vi "Cancella Celle.vi"(0 "report in":T1, 7 "start (-1, -1)":cluster{"row":i32, "column":i32}={"row"=-1, "column"=-1}, 9 "end (-1, -1)":cluster{"row":i32, "column":i32}={"row"=-1, "column"=-1}, 11 "error in (no error)":errorcluster, 12 "name (\"\")":string) -> (4 "report out":T1, 15 "error out":errorcluster)   [LabVIEW 2022 SP3]
doc: "Merges the range of cells specified by the start and end clusters."
uses:
  <vilib>/Utility/NIReport.llb/NI_ReportGenerationCore.lvlib
  <vilib>/Utility/NIReport.llb/NI_report.lvclass
  <vilib>/Utility/NIReport.llb/Generate Report Object Reference.ctl
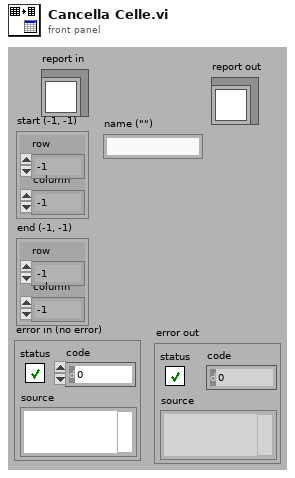
[diagram p1: front panel]
types:
  T1 = typedef "Generate Report Object Reference.ctl" = refnum<class "NI_report.lvclass">
  T2 = typedef "Generate Report Data Members.ctl" = cluster{"Title Text":string, "Header Text":string, "Body Text":string, "Footer Text":string, "Image List":path[], "NIReports.Report":refnum<k7>, "Report Type":enum16{"Standard Report", "HTML", "Word", "Excel"}, "Font Tag":string, "Word._Application":refnum<k7>, "Word._Document":refnum<k7>, "Word.Documents":refnum<k7>, "Word.InlineShapes":refnum<k7>, "Word.Tables":refnum<k7>, "Excel._Application":refnum<k7>, "Excel._Workbook":refnum<k7>, "Excel._Worksheet":refnum<k7>, "Excel.Sheets":refnum<k7>, "Excel.Shapes":refnum<k7>, "font":T3, "application directory":path}
  T3 = typedef "font.ctl" = cluster{"font name":string, "font size":dbl, "bold":u16, "italic":u16, "underline":u16, "strike through":u16, "font color":u32}
  T4 = typedef "Generate Report Object Reference.ctl" = refnum<k1>
  T5 = enum16{"Standard Report", "HTML", "Word", "Excel"}
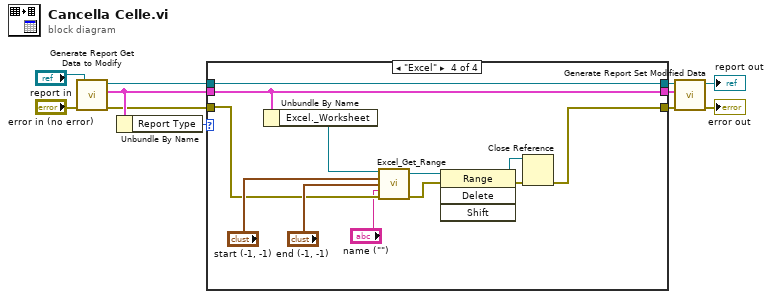
[diagram p0: block diagram]
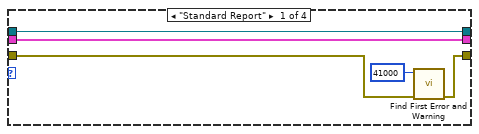
[diagram p2: hidden frame]
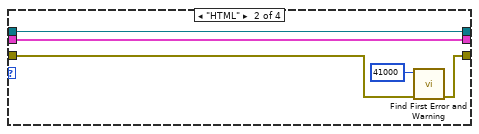
[diagram p3: hidden frame]
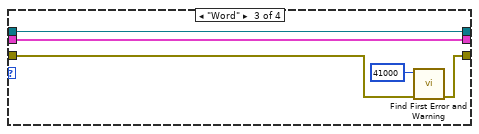
[diagram p4: hidden frame]
diagram:
  n1 = call <vilib>:"Generate Report Get Data to Modify.vi"("error in (no error)"="error in (no error)", "report in"="report in") -> ("error out"=w4:errorcluster, "data"=w9:T2, "report out"=w7:T4)  [unwired: 2 in, 1 out]
  n2 = Unbundle By Name(w9) -> ("Report Type"=w3:T5)
  n3 = case shown="\"Excel\"" w3 {
    tunnel: w4 -> [w13 w18 w23 w30]
    tunnel: w7 -> [w16 w21 w26 w38]
    tunnel: [w16 w21 w26 w38] -> w8
    tunnel: w9 -> [w15 w20 w25 w37]
    tunnel: [w15 w20 w25 w37] -> w10
    tunnel: [w12 w17 w22 w36] -> w11
    frame "Standard Report" {
      n4 = call <vilib>:"Find First Error and Warning.vi"("error in (no error)"=w13, "error code"=41000) -> ("error out"=w12:errorcluster)  [unwired: 4 in, 1 out]
    }
    frame "HTML" {
      n5 = call <vilib>:"Find First Error and Warning.vi"("error in (no error)"=w18, "error code"=41000) -> ("error out"=w17:errorcluster)  [unwired: 4 in, 1 out]
    }
    frame "Word" {
      n6 = call <vilib>:"Find First Error and Warning.vi"("error in (no error)"=w23, "error code"=41000) -> ("error out"=w22:errorcluster)  [unwired: 4 in, 1 out]
    }
    frame "Excel" {
      n7 = Unbundle By Name(w37) -> ("Excel._Worksheet"=w33:refnum<k7>)
      n8 = call "Excel_Get_Range.vi"("Excel._Worksheet"=w33, "start"="start (-1, -1)", "end"="end (-1, -1)", "name"="name (\"\")", "error out 2"=w30) -> ("Range"=w29:refnum<k7>, "error out"=w28:errorcluster)  [unwired: 9 in]
      n9 = invoke class="Range" method="Delete"(reference=w29, error in=w28) -> (reference out=w34:refnum<k7>, error out=w35:errorcluster)  [unwired: 2 in, 2 out]
      n10 = Close Reference(reference=w34, error in (no error)=w35) -> (error out=w36:errorcluster)
    }
  }
  n11 = call <vilib>:"Generate Report Set Modified Data.vi"("error in (no error)"=w11, "data"=w10, "report in"=w8) -> ("error out"=→"error out":errorcluster, "report out"=→"report out":T4)  [unwired: 3 in]
